vi "SVN_Checkout.vi"(6 "checkout? (T)":bool=TRUE, 7 "Path":string, 8 "error in (no error)":errorcluster, 9 "URL":string, 10 "Password":string, 11 "Username":string) -> (0 "error out":errorcluster, 1 "command":string, 2 "standard output":string, 3 "standard error":string)   [LabVIEW 2017]
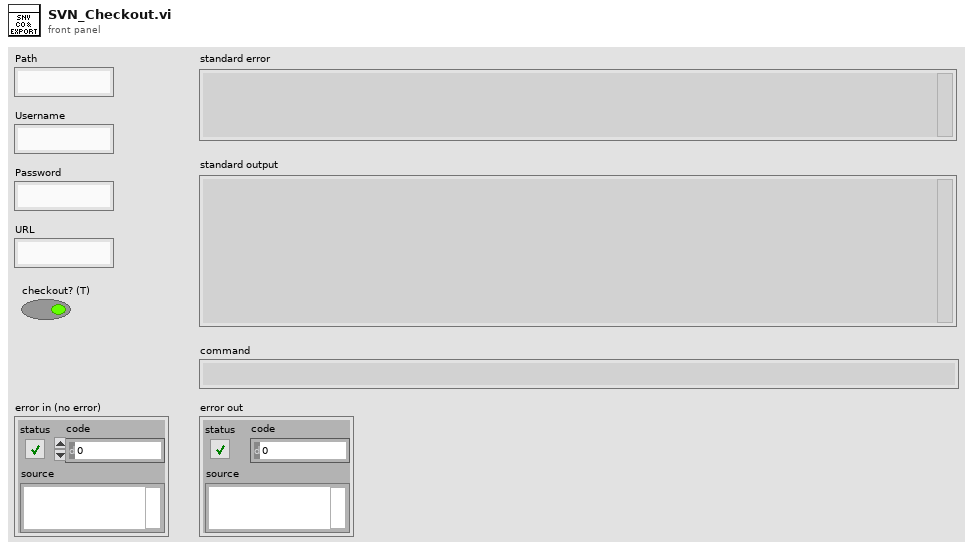
[diagram p1: front panel]
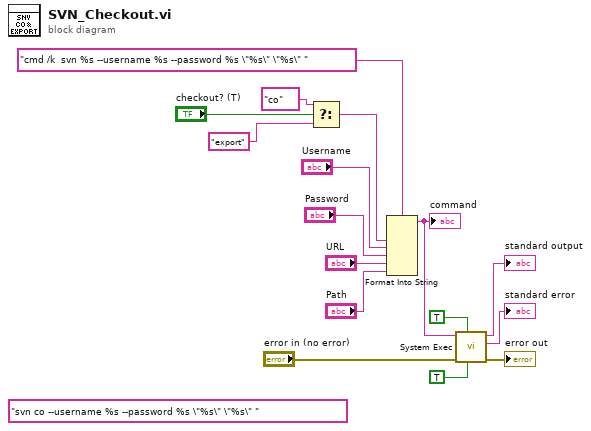
[diagram p0: block diagram]
diagram:
  (unwired) "svn co --username %s --password %s \"%s\" \"%s\" "
  n1 = Select(t="co", s="checkout? (T)", f="export") -> (s? t:f=w1:string)
  n2 = Format Into String(format string="cmd /k  svn %s --username %s --password %s \"%s\" \"%s\" ", w1, "Username", "Password", "URL", "Path") -> (resulting string=w10:string)  [unwired: 2 in, 1 out]
  "command" <- w10
  n3 = call <vilib>:"System Exec.vi"("run minimized? (F)"=TRUE, "wait until completion? (T)"=TRUE, "error in (no error)"="error in (no error)", "command line"=w10) -> ("error out"=→"error out":errorcluster, "standard error"=→"standard error":string, "standard output"=→"standard output":string)  [unwired: 4 in, 1 out]
